vi "Read MTi Gyro.vi"(8 "error in (no error)":errorcluster, 11 "Supervisor in":refnum<class "Supervisor.lvclass">) -> (0 "error out":errorcluster, 2 "MTi Gyro":bool=TRUE, 3 "Supervisor out":refnum<class "Supervisor.lvclass">)   [LabVIEW 2014, in "Supervisor.lvclass"]
uses:
  Supervisor.lvclass
  Supervisor.lvclass/Supervisor.ctl
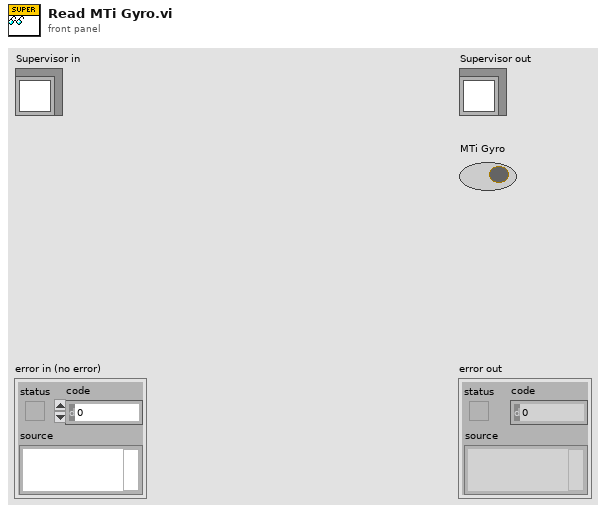
[diagram p1: front panel]
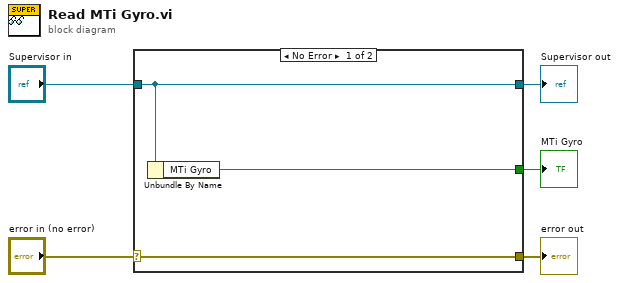
[diagram p0: block diagram]
diagram:
  n1 = case shown="No Error" "error in (no error)" {
    selector: "error in (no error)" -> [w8 w9]
    tunnel: [w8 w9] -> w4
    tunnel: [w7 w10] -> w2
    tunnel: "Supervisor in" -> [w7 w10]
    tunnel: [w6 _] -> w1
    frame No Error {
      n2 = Unbundle By Name(w7) -> ("MTi Gyro"=w6:bool)
    }
    frame Error {
    }
  }
  "error out" <- w4
  "Supervisor out" <- w2
  "MTi Gyro" <- w1
